vi "Actor Core.vi"(8 "error in":errorcluster, 11 "Application Actor":refnum<class "Application Actor.lvclass">) -> (0 "error out":errorcluster, 3 "Application Actor out":refnum<class "Actor.lvclass">)   [LabVIEW 2018, in "Application Actor.lvlib" / "Application Actor.lvclass"]
doc: "This is Actor Core.vi, the main message handling loop for Actors. An actor usually just sits in this loop and processes messages as they arrive. Any error returned by the message Do.vi call will stop the loop, with error code 43 as the canonical signal to stop with no error sent to caller. Descendants may override that in Handle Error.vi.\n\nThe VI Properties of this VI take care of opening the panel when this VI is called and closing it again when it finishes execution.e"
uses:
  Application Actor.lvclass
  C:/Program Files (x86)/National Instruments/LabVIEW 2018/vi.lib/ActorFramework/Actor/Actor.lvclass
  <vilib>/ActorFramework/Actor/Actor.lvclass
  Alpha Actor/Alpha/Alpha.lvclass
  Beta Actor/Beta/Beta.lvclass
  <vilib>/ActorFramework/Actor/Actor.lvclass/Actor.ctl
  <vilib>/ActorFramework/Message Enqueuer/Message Enqueuer.lvclass/Message Enqueuer.ctl
  Application Actor.lvclass/Application Actor.ctl
  <vilib>/ActorFramework/Message Enqueuer/Init from Existing Queue.vi
  <vilib>/ActorFramework/Message Enqueuer/Enqueue.vi
  <vilib>/ActorFramework/Stop Msg/Stop Msg.lvclass
  C:/Program Files (x86)/National Instruments/LabVIEW 2018/vi.lib/ActorFramework/Message/Message.lvclass
  <vilib>/ActorFramework/Message Priority Queue/Priority Enqueue.vi
  <vilib>/ActorFramework/Message Enqueuer/Message Enqueuer.lvclass
panel:
  in  "stop signal":bool
  out "Event Log":string
  in  "Stop":bool
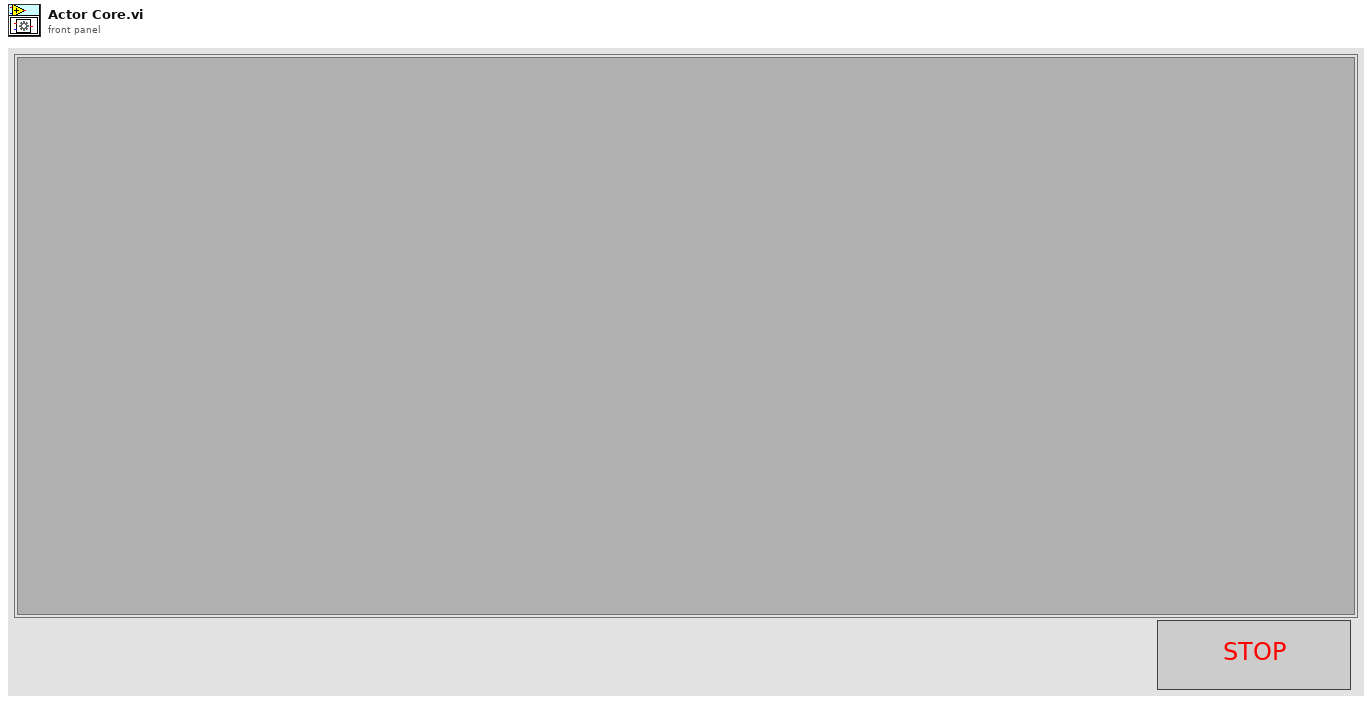
[diagram p1: front panel]
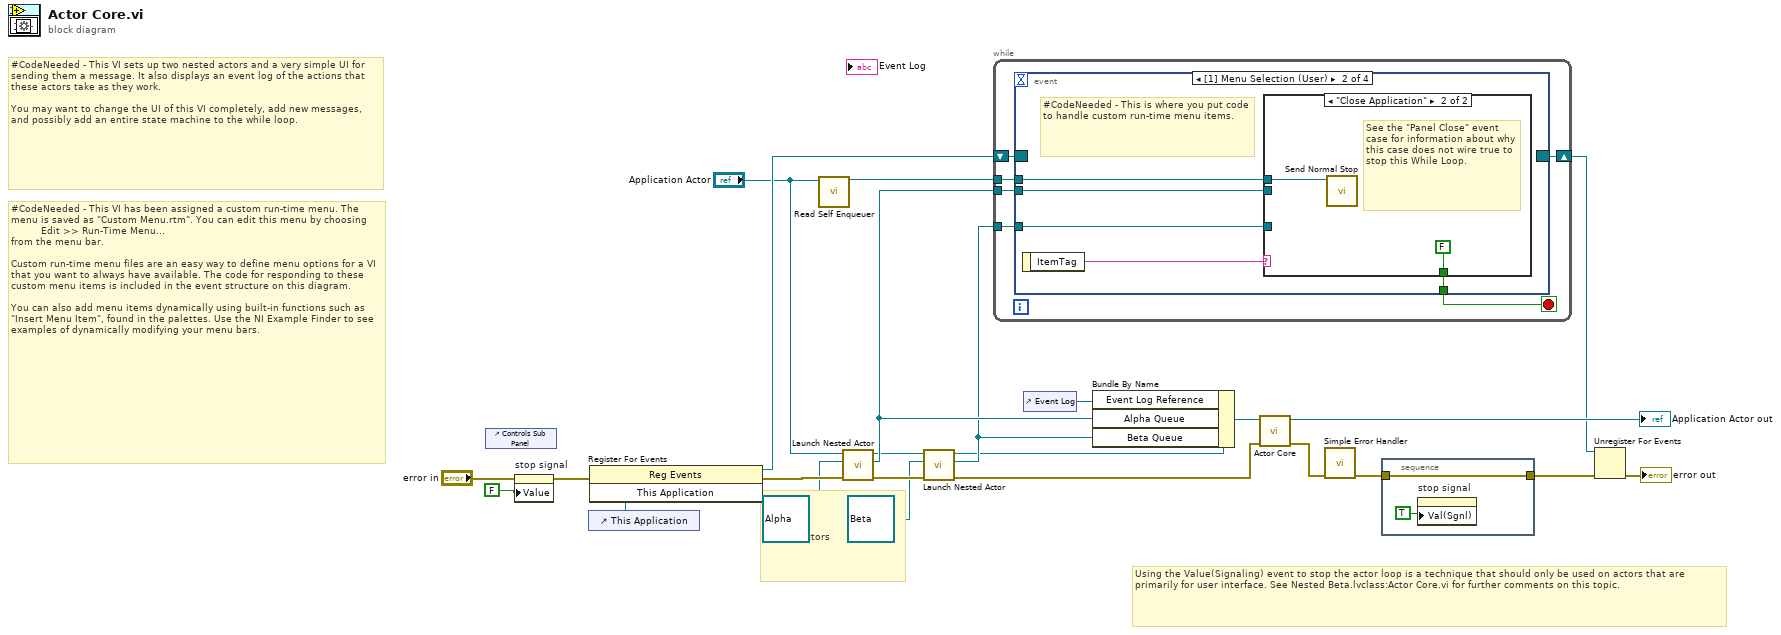
[diagram p0: block diagram]
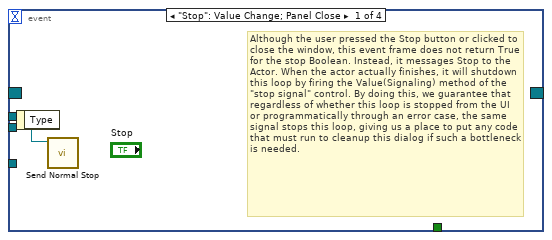
[diagram p2: hidden frame]
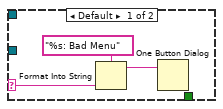
[diagram p3: hidden frame]
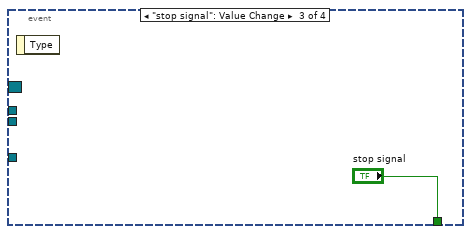
[diagram p4: hidden frame]
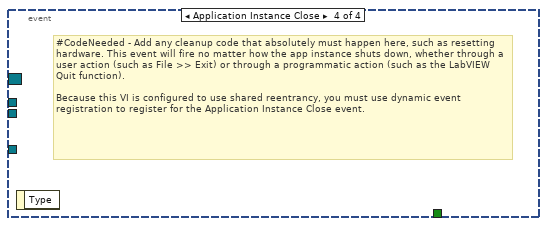
[diagram p5: hidden frame]
diagram:
  # "#CodeNeeded - This VI has been assigned a custom run-time menu. The menu is saved as \"Custom Menu.rtm\". You can edit this menu by choosing \n          Edit >> Run-Time Menu...\nfrom the menu bar.\n\nCustom run-time menu files are an easy way to define menu options for a VI that you want to always have available. The code for responding to these custom menu items is included in the event structure on this diagram.\n\nYou can also add menu items dynamically using built-in functions such as \"Insert Menu Item\", found in the palettes. Use the NI Example Finder to see examples of dynamically modifying your menu bars."
  # "Using the Value(Signaling) event to stop the actor loop is a technique that should only be used on actors that are primarily for user interface. See Nested Beta.lvclass:Actor Core.vi for further comments on this topic."
  # "#CodeNeeded - This VI sets up two nested actors and a very simple UI for sending them a message. It also displays an event log of the actions that these actors take as they work. \n\nYou may want to change the UI of this VI completely, add new messages, and possibly add an entire state machine to the while loop."
  # "Nested actors"
  n1 = control-ref of="Controls Sub Panel"() -> ()  [unwired: 1 out]
  n2 = property on="stop signal" class="Bool (strict)"(error in="error in", "Value"=FALSE ("stop")) -> (error out=w9:errorcluster)  [unwired: 1 in, 1 out]
  n3 = control-ref of="This Application"() -> (w7:refnum<vi>)
  n4 = register-events(error in=w9, w7) -> (reference out=w13:refnum<event-registration>, error out=w8:errorcluster)  [unwired: 1 in]
  n5 = call <vilib>:"Read Self Enqueuer.vi"("Actor"="Application Actor") -> ("Self Enqueuer"=w19:refnum<class "Message Enqueuer.lvclass">)  [unwired: 10 in]
  n6 = call <vilib>:"Launch Nested Actor.vi"("error in (no error)"=w8, "Nested Actor"=refnum<class "Alpha.lvclass"> refnum ("Alpha.lvclass"), "Caller Actor in"="Application Actor") -> ("error out"=w23:errorcluster, "Nested Actor's Enqueuer"=w18:refnum<class "Message Enqueuer.lvclass">, "Caller Actor out"=w5:refnum<class "Application Actor.lvclass">)  [unwired: 6 in]
  n7 = call <vilib>:"Launch Nested Actor.vi"("error in (no error)"=w23, "Nested Actor"=refnum<class "Beta.lvclass"> refnum ("Beta.lvclass"), "Caller Actor in"=w5) -> ("error out"=w22:errorcluster, "Nested Actor's Enqueuer"=w17:refnum<class "Message Enqueuer.lvclass">, "Caller Actor out"=w2:refnum<class "Application Actor.lvclass">)  [unwired: 6 in]
  n8 = while {
    tunnel: w19 -> [w30]
    tunnel: w18 -> [w29]
    tunnel: w17 -> [w28]
    shift-right: [w25] -> w12
    shift-left: w13 -> [w26]
    stop <- w27 stop-if-true
    n9 = event shown="[1] Menu Selection (User)" {
      selector: w26 -> [_ _ _ _]
      dyn-events: [_ _ _ _] -> w25
      timeout: _ -> [_ _ _ _]
      tunnel: w30 -> [w31 w33 _ _]
      tunnel: w29 -> [_ w35 _ _]
      tunnel: w28 -> [_ w34 _ _]
      tunnel: [_ w32 "stop signal" _] -> w27
      event "Stop": Value Change; Panel Close {
        # "Although the user pressed the Stop button or clicked to close the window, this event frame does not return True for the stop Boolean. Instead, it messages Stop to the Actor. When the actor actually finishes, it will shutdown this loop by firing the Value(Signaling) method of the \"stop signal\" control. By doing this, we guarantee that regardless of whether this loop is stopped from the UI or programmatically through an error case, the same signal stops this loop, giving us a place to put any code that must run to cleanup this dialog if such a bottleneck is needed."
        n10 = event-data() -> ()  [unwired: 1 in, 1 out]
        n11 = call <vilib>:"Send Normal Stop.vi"("Message Enqueuer"=w31) -> ()  [unwired: 10 in, 1 out]
      }
      event Menu Selection (User) {
        # "#CodeNeeded - This is where you put code to handle custom run-time menu items."
        n12 = event-data() -> ("ItemTag"=w36:string)  [unwired: 1 in]
        n13 = case shown="\"Close Application\"" w36 {
          selector: w36 -> [w39 _]
          tunnel: w35 -> [_ _]
          tunnel: w34 -> [_ _]
          tunnel: w33 -> [_ w41]
          tunnel: [_ FALSE] -> w32
          frame Default {
            n14 = Format Into String(format string="%s: Bad Menu" ("Unlocalized"), w39) -> (resulting string=w38:string)  [unwired: 2 in, 1 out]
            n15 = One Button Dialog(message=w38) -> ()  [unwired: 1 in, 1 out]
          }
          frame "Close Application" {
            # "See the \"Panel Close\" event case for information about why this case does not wire true to stop this While Loop."
            n16 = call <vilib>:"Send Normal Stop.vi"("Message Enqueuer"=w41) -> ()  [unwired: 10 in, 1 out]
          }
        }
      }
      event "stop signal": Value Change {
        n17 = event-data() -> ()  [unwired: 1 in, 1 out]
      }
      event Application Instance Close {
        # "#CodeNeeded - Add any cleanup code that absolutely must happen here, such as resetting hardware. This event will fire no matter how the app instance shuts down, whether through a user action (such as File >> Exit) or through a programmatic action (such as the LabVIEW Quit function).\n\nBecause this VI is configured to use shared reentrancy, you must use dynamic event registration to register for the Application Instance Close event."
        n18 = event-data() -> ()  [unwired: 1 in, 1 out]
      }
    }
  }
  n19 = control-ref of="Event Log"() -> (w20:refnum<vi>)
  n20 = Bundle By Name(cluster=w2, "Event Log Reference"=w20, "Alpha Queue"=w18, "Beta Queue"=w17) -> (w21:refnum<class "Application Actor.lvclass">)
  n21 = call-parent "Actor Core.vi"("error in"=w22, "Actor in"=w21) -> ("error out"=w15:errorcluster, "Actor out"=→"Application Actor out":refnum<class "Actor.lvclass">)  [unwired: 8 in]
  n22 = call <vilib>:"Simple Error Handler.vi"("error in (no error)"=w15) -> ("error out"=w14:errorcluster)  [unwired: 4 in, 4 out]
  n23 = stacked-sequence {
    tunnel: [w43] -> w11
    tunnel: w14 -> [w43]
    frame #0 {
      n24 = property on="stop signal" class="Bool (strict)"("Val(Sgnl)"=TRUE ("stop")) -> ()  [unwired: 2 in, 2 out]
    }
  }
  n25 = Unregister For Events(event registration refnum=w12, error in=w11) -> (error out=→"error out":errorcluster)
